vi "New Edit Element.vi"(8 "error in (no error)":errorcluster, 11 "Product-B in":refnum<class "Product-B.lvclass">) -> (0 "error out":errorcluster, 3 "Product-B out":refnum<class "Product-B.lvclass">)   [LabVIEW 2018, in "Product-B.lvclass"]
uses:
  Product-B.lvclass
  <vilib>/Utility/error.llb/Error Cluster From Error Code.vi
  <vilib>/ErrorRing/Error Ring.xnode
  U:/modules/labview-orm/demo/Product.lvclass
  U:/modules/labview-orm/_Serializable Base Object/_ISerializable.lvclass
panel:
  in  "Current":dbl format="%.5g"
  in  "Voltage":dbl format="%.5g"
  in  "cancel button":bool
  in  "ok button":bool
  in  "isObsolete":bool
  in  "status":u8
  in  "mayExplode":bool
  in  "Power":dbl format="%.5g"
  out "uid":u64
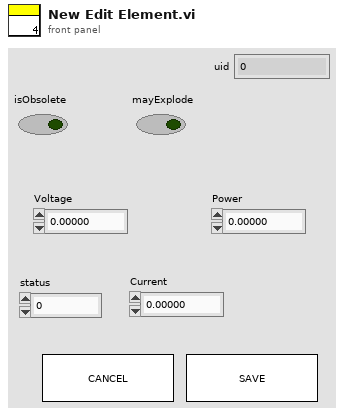
[diagram p1: front panel]
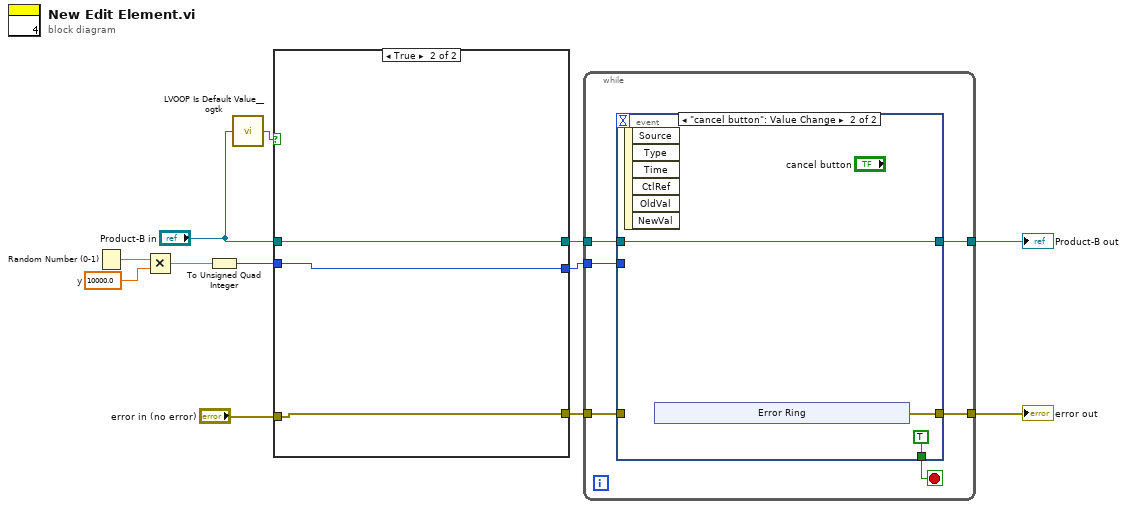
[diagram p0: block diagram]
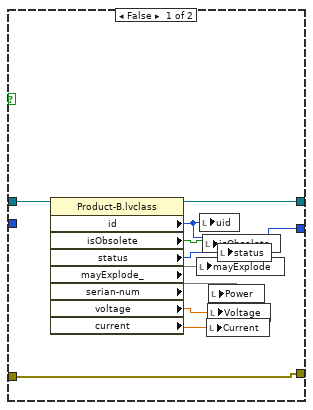
[diagram p2: hidden frame]
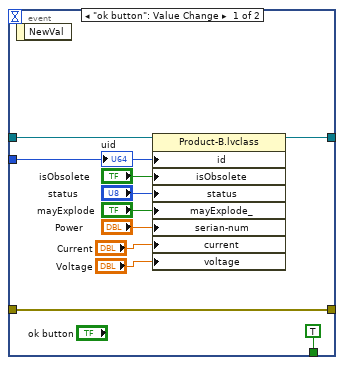
[diagram p3: hidden frame]
diagram:
  w11 = 10000.0  # y
  n1 = Random Number (0-1)() -> (number: 0 to 1=w12:dbl)
  n2 = Multiply(x=w12, y=w11) -> (x*y=w10:dbl)
  n3 = To Unsigned Quad Integer(1:w10) -> (0:w6:u64)
  n4 = call <userlib>:"LVOOP Is Default Value__ogtk.vi"("Object"="Product-B in") -> ("Is Default Value?"=w7:bool)
  n5 = case shown="True" w7 {
    tunnel: "Product-B in" -> [w22 w23]
    tunnel: [w21 w23] -> w9
    tunnel: [w20 w25] -> w8
    tunnel: "error in (no error)" -> [w20 w25]
    tunnel: w6 -> [_ w24]
    tunnel: [w19 w24] -> w5
    frame False {
      n6 = property class="Product-B.lvclass"(reference=w22) -> (reference out=w21:refnum<class "Product-B.lvclass">, "id"=w19:i32, "isObsolete"=w16:bool, "status"=w17:u8, "mayExplode_"=w18, "serian-num"=w15, "voltage"=w14:sgl, "current"=w13:dbl)  [unwired: 1 in, 1 out]
      n7 = local write "mayExplode"(w18) -> ()
      n8 = local write "uid"(w19) -> ()
      n9 = local write "isObsolete"(w16) -> ()
      n10 = local write "Current"(w13) -> ()
      n11 = local write "Voltage"(w14) -> ()
      n12 = local write "Power"(w15) -> ()
      n13 = local write "status"(w17) -> ()
    }
    frame True {
    }
  }
  n14 = while {
    tunnel: w8 -> [w28]
    tunnel: w9 -> [w31]
    tunnel: [w30] -> w3
    tunnel: [w29] -> w1
    tunnel: w5 -> [w26]
    stop <- w27 stop-if-true
    n15 = event shown="[1] \"cancel button\": Value Change" {
      selector: _ -> [_ _]
      dyn-events: _ -> [_ _]
      timeout: _ -> [_ _]
      tunnel: w31 -> [w42 w45]
      tunnel: [w41 w45] -> w30
      tunnel: [w40 w44] -> w29
      tunnel: w28 -> [w40 _]
      tunnel: [TRUE TRUE] -> w27
      tunnel: w26 -> [w38 _]
      event "ok button": Value Change {
        n16 = event-data() -> ()  [unwired: 1 in, 1 out]
        n17 = property class="Product-B.lvclass"(reference=w42, "id"=w38, "isObsolete"="isObsolete", "status"="status", "mayExplode_"="mayExplode", "serian-num"="Power", "current"="Current", "voltage"="Voltage") -> (reference out=w41:refnum<class "Product-B.lvclass">)  [unwired: 1 in, 1 out]
        "uid" <- w38
      }
      event "cancel button": Value Change {
        n18 = event-data() -> ()  [unwired: 1 in, 6 out]
        n19 = xnode "Error Ring"() -> ("error out"=w44:errorcluster)
      }
    }
  }
  "error out" <- w1
  "Product-B out" <- w3
